vi "GetDistWithDispDotSpan.vi"(8 "错误输入（无错误）":errorcluster, 9 "闸门序号":i32, 10 "显示点间隔":u16, 11 "需要转换的通道":u8) -> (0 "错误输出":errorcluster, 3 "返回值":sgl)   [LabVIEW 2014]
uses:
  ZXUTConfigMgr.dll
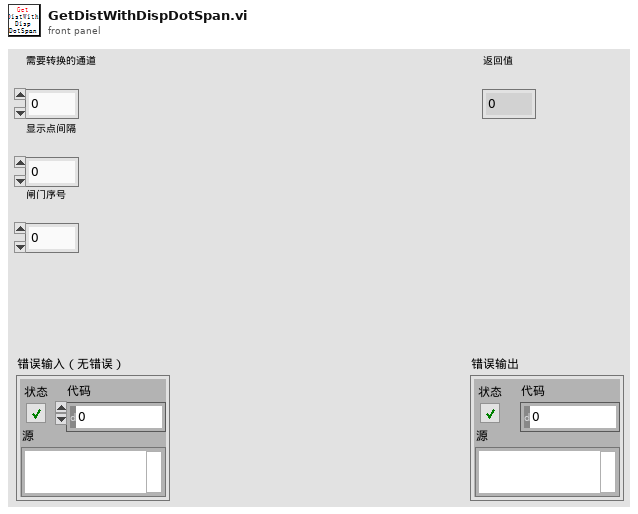
[diagram p1: front panel]
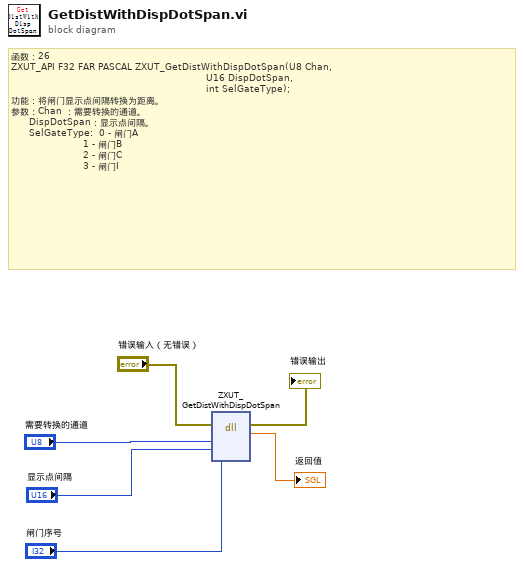
[diagram p0: block diagram]
diagram:
  # "函数：26\nZXUT_API F32\tFAR PASCAL ZXUT_GetDistWithDispDotSpan(U8 Chan, \n                                                                 U16 DispDotSpan,\n                                                                 int SelGateType);\n功能：将闸门显示点间隔转换为距离。\n参数：Chan ：需要转换的通道。\n      DispDotSpan：显示点间隔。\n      SelGateType:  0 - 闸门A \n                        1 - 闸门B\n                        2 - 闸门C\n                        3 - 闸门I"
  n1 = dll-call lib="PTH2eabs D软件超声实时监测软件ZXUTAppDemo(华南理工V02.00)X86DllZXUTConfigMgr.dll" fn="ZXUT_GetDistWithDispDotSpan"(error in="错误输入（无错误）", "Chan"="需要转换的通道", "DispDotSpan"="显示点间隔", "SelGateType"="闸门序号") -> (error out=→"错误输出":errorcluster, "返回值"=→"返回值":sgl)  [unwired: 5 in, 1 out]
